vi "Write Gannt Chart.vi"(8 "error in (no error)":errorcluster, 10 "Gannt Chart":T1[][](array[typedef]), 11 "GanntChart in":refnum<class "GanntChart.lvclass">) -> (0 "error out":errorcluster, 3 "GanntChart out":refnum<class "GanntChart.lvclass">)   [LabVIEW 2013, in "GanntChart.lvclass"]
uses:
  GanntChart.lvclass
  Controls/GanntChart_Element.ctl
  GanntChart.lvclass/GanntChart.ctl
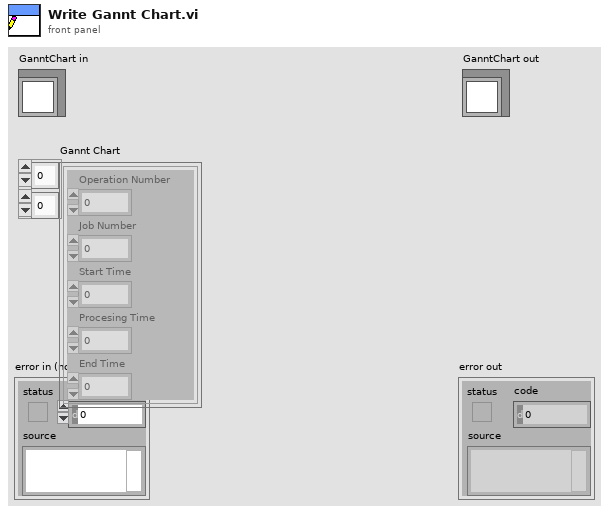
[diagram p1: front panel]
types:
  T1 = typedef "GanntChart_Element.ctl" = cluster{"Operation Number":i32, "Job Number":i32, "Start Time":i32, "Procesing Time":u16, "End Time":i32}
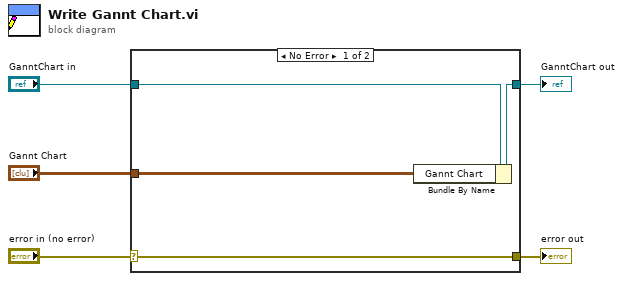
[diagram p0: block diagram]
diagram:
  n1 = case shown="No Error" "error in (no error)" {
    selector: "error in (no error)" -> [w9 w10]
    tunnel: [w9 w10] -> w4
    tunnel: [w7 w11] -> w2
    tunnel: "GanntChart in" -> [w8 w11]
    tunnel: "Gannt Chart" -> [w6 _]
    frame No Error {
      n2 = Bundle By Name(cluster=w8, "Gannt Chart"=w6) -> (w7:refnum<class "GanntChart.lvclass">)
    }
    frame Error {
    }
  }
  "error out" <- w4
  "GanntChart out" <- w2
